vi "create population index.vi"(11 "deaths global csv array":string[][](array[string])) -> (2 "Populations":i32[](array[numeric]), 3 "Name and populations cluster":cluster{string, i32}[](array[cluster]))   [LabVIEW 2019]
uses:
  <vilib>/httpClient/LabVIEWHTTPClient.lvlib
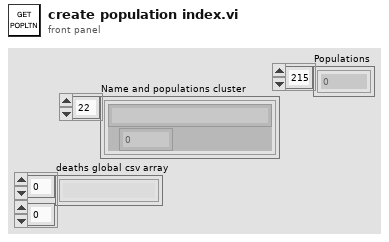
[diagram p1: front panel]
types:
  T1 = typedef "LabVIEWHTTPClient.lvlib/ClientHandle.ctl" = refnum<k1>
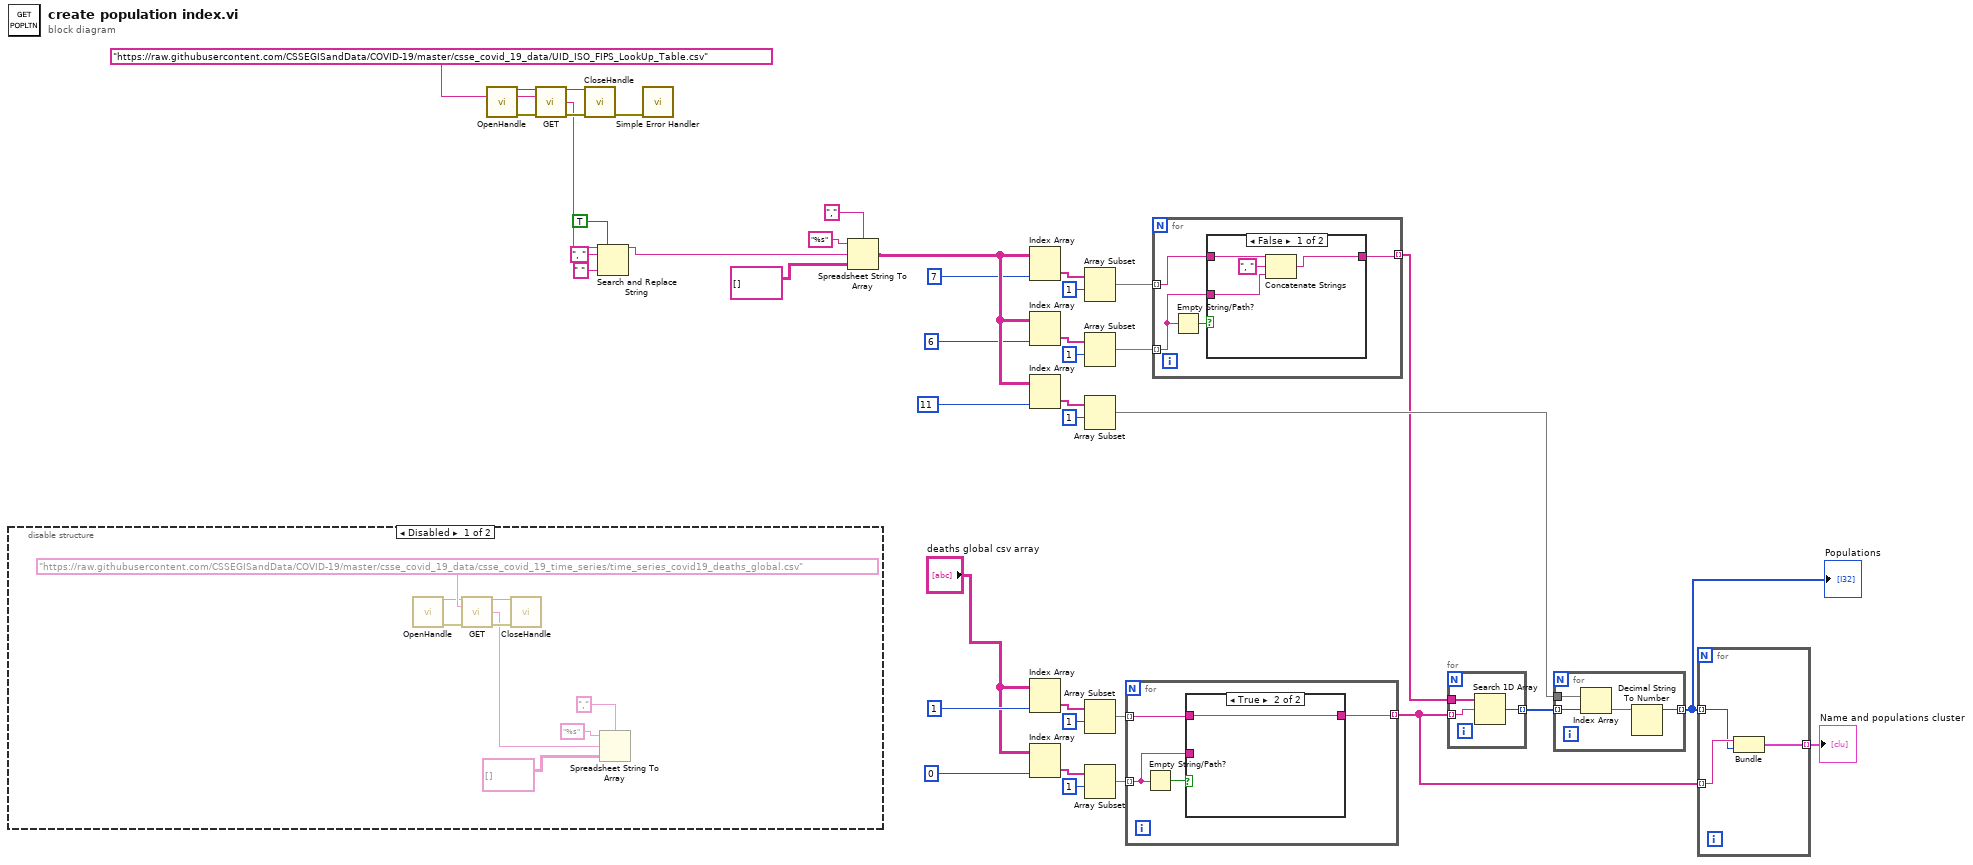
[diagram p0: block diagram]
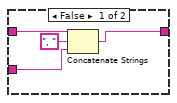
[diagram p4: hidden frame]
diagram:
  n1 = disable-structure shown="Disabled" {
    frame Disabled {
      n2 = call <vilib>:"OpenHandle.vi"() -> ("client handle out"=w43:T1, "error out"=w44:errorcluster)  [unwired: 14 in]
      n3 = call <vilib>:"GET.vi"("client handle"=w43, "url"="https://raw.githubusercontent.com/CSSEGISandData/COVID-19/master/csse_covid_19_data/csse_covid_19_time_series/time_series_covid19_deaths_global.csv", "error in (no error)"=w44) -> ("client handle out"=w46:T1, "body"=w42:string, "error out"=w45:errorcluster)  [unwired: 9 in, 1 out]
      n4 = call <vilib>:"CloseHandle.vi"("client handle"=w46, "error in (no error)"=w45) -> ()  [unwired: 13 in, 1 out]
      n5 = Spreadsheet String To Array(delimiter (Tab)=",", format string="%s", spreadsheet string=w42, array type (2D Dbl)=string[][] []) -> ()  [unwired: 1 out]
    }
    frame Enabled {
    }
  }
  n6 = call <vilib>:"OpenHandle.vi"() -> ("client handle out"=w23:T1, "error out"=w22:errorcluster)  [unwired: 14 in]
  n7 = call <vilib>:"GET.vi"("client handle"=w23, "url"="https://raw.githubusercontent.com/CSSEGISandData/COVID-19/master/csse_covid_19_data/UID_ISO_FIPS_LookUp_Table.csv", "error in (no error)"=w22) -> ("client handle out"=w20:T1, "body"=w7:string, "error out"=w21:errorcluster)  [unwired: 9 in, 1 out]
  n8 = call <vilib>:"CloseHandle.vi"("client handle"=w20, "error in (no error)"=w21) -> ("error out"=w1:errorcluster)  [unwired: 13 in]
  n9 = Search and Replace String(replace all?=TRUE ("replace all? (F)"), input string=w7, search string=", ", replace string=" " ("replace string (\"\")")) -> (result string=w3:string)  [unwired: 4 in, 3 out]
  n10 = call <vilib>:"Simple Error Handler.vi"("error in (no error)"=w1) -> ()  [unwired: 4 in, 5 out]
  n11 = Spreadsheet String To Array(delimiter (Tab)=",", format string="%s", spreadsheet string=w3, array type (2D Dbl)=string[][] []) -> (array=w33:string[][])
  n12 = Index Array(array=w33, index (col)=7 ("disabled index (col)")) -> (element=w28:string[])  [unwired: 1 in]
  n13 = Index Array(array=w33, index (col)=6 ("disabled index (col)")) -> (element=w25:string[])  [unwired: 1 in]
  n14 = Index Array(array=w33, index (col)=11 ("disabled index (col)")) -> (element=w31:string[])  [unwired: 1 in]
  n15 = Index Array(array="deaths global csv array", index (col)=1 ("disabled index (col)")) -> (element=w9:string[])  [unwired: 1 in]
  n16 = Index Array(array="deaths global csv array", index (col)=0 ("disabled index (col)")) -> (element=w13:string[])  [unwired: 1 in]
  n17 = Array Subset(array=w28, index=1) -> (w34:string[])  [unwired: 1 in]
  n18 = Array Subset(array=w25, index=1) -> (w35:string[])  [unwired: 1 in]
  n19 = Array Subset(array=w31, index=1) -> (w37:string[])  [unwired: 1 in]
  n20 = Array Subset(array=w9, index=1) -> (w11:string[])  [unwired: 1 in]
  n21 = Array Subset(array=w13, index=1) -> (w15:string[])  [unwired: 1 in]
  n22 = for {
    tunnel: w11 -> [w54] mode=indexing
    tunnel: w15 -> [w52] mode=indexing
    tunnel: [w51] -> w40 mode=indexing
    n23 = Empty String/Path?(string/path=w52) -> (empty?=w53:bool)
    n24 = case shown="True" w53 {
      tunnel: w54 -> [w58 w59]
      tunnel: [w55 w59] -> w51
      tunnel: w52 -> [w56 _]
      frame False {
        n25 = Concatenate Strings(w58, ", " ("string"), w56) -> (w55:string)
      }
      frame True {
      }
    }
  }
  n26 = for {
    tunnel: w34 -> [w63] mode=indexing
    tunnel: w35 -> [w61] mode=indexing
    tunnel: [w60] -> w36 mode=indexing
    n27 = Empty String/Path?(string/path=w61) -> (empty?=w62:bool)
    n28 = case shown="False" w62 {
      tunnel: w63 -> [w67 w68]
      tunnel: [w64 w68] -> w60
      tunnel: w61 -> [w65 _]
      frame False {
        n29 = Concatenate Strings(w67, ", " ("string"), w65) -> (w64:string)
      }
      frame True {
      }
    }
  }
  n30 = for {
    tunnel: w36 -> [w71]
    tunnel: w40 -> [w70] mode=indexing
    tunnel: [w69] -> w38 mode=indexing
    n31 = Search 1D Array(1D array=w71, element=w70) -> (index of element=w69:i32)  [unwired: 1 in]
  }
  n32 = for {
    tunnel: w38 -> [w75] mode=indexing
    tunnel: [w72] -> w39 mode=indexing
    tunnel: w37 -> [w73]
    n33 = Index Array(array=w73, index=w75) -> (element=w74:string)
    n34 = Decimal String To Number(string=w74) -> (number=w72:i32)  [unwired: 2 in, 1 out]
  }
  "Populations" <- w39
  n35 = for {
    tunnel: w39 -> [w77] mode=indexing
    tunnel: w40 -> [w78] mode=indexing
    tunnel: [w76] -> w41 mode=indexing
    n36 = Bundle(w78, w77) -> (w76:cluster{string, i32})  [unwired: 1 in]
  }
  "Name and populations cluster" <- w41
